vi "LabVIEW to Formula.vi"(11 "output ref":refnum<vi>) -> (3 "element":string)   [LabVIEW 2018, in "RPN.lvlib"]
uses:
  RPN.lvlib
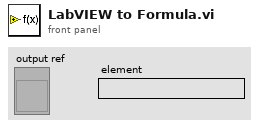
[diagram p1: front panel]
types:
  T1 = typedef "RPN.lvlib/Node Type Def.ctl" = cluster{"Class Name":string, "Label":string, "Value":variant, "Arity":u8}
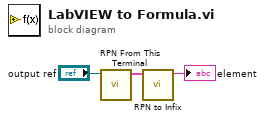
[diagram p0: block diagram]
diagram:
  n1 = call "RPN From This Terminal.vi"("output ref"="output ref") -> ("Array"=w2:T1[])  [unwired: 10 in]
  n2 = call "RPN to Infix.vi"("Array 2"=w2) -> ("element"=→"element":string)  [unwired: 10 in]
